vi "Enumerate Connected IMAQdx DirectShow Cameras.vi"() -> ()   [LabVIEW 2011]
uses:
  <vilib>/vision/driver/NI_Vision_Acquisition_Software.lvlib
panel:
  out "Connected Camera Interface name":string[](array[string])
  out "IMAQdx Open Camera error":errorcluster[](array[cluster])
  out "IMAQdx Enumerate Connected Only Cameras Camera Information Array":T1(array[cluster]) {"BusType" format="%x"; "SerialNumberLow" format="%.0x"; "SerialNumberHigh" format="%.0x"}
  # "Certain USB DirectShow cameras will always as connected when they are not.  Acording to one vendor :\n\"USB cameras that implement their DirectShow driver as a data source filter and register the filter as a \"video capture device\" \nwill always shows the device (filter) no matter whether the physical device is connected or not. \nThis contrasts with many other USB cameras (e.g. all web cameras) which implement their DirectShow support with a WDM stream driver.\""
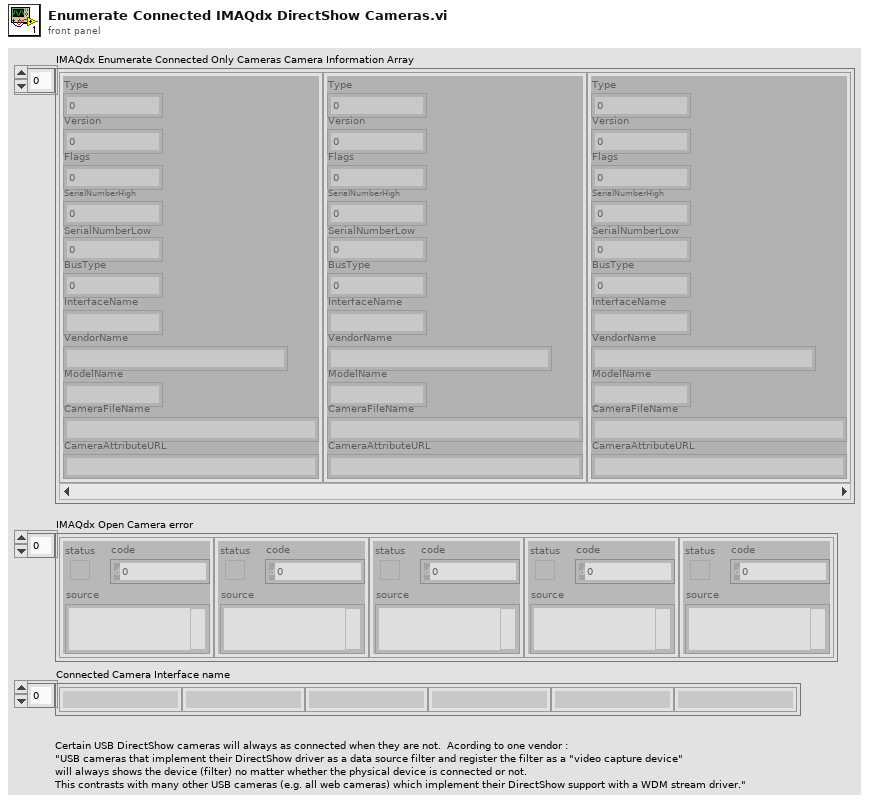
[diagram p1: front panel]
types:
  T1 = cluster{"Type":u32, "Version":u32, "Flags":u32, "SerialNumberHigh":u32, "SerialNumberLow":u32, "BusType":u32, "InterfaceName":string, "VendorName":string, "ModelName":string, "CameraFileName":string, "CameraAttributeURL":string}[]
  T2 = typedef "IMAQdx.ctl" = refnum<k21>
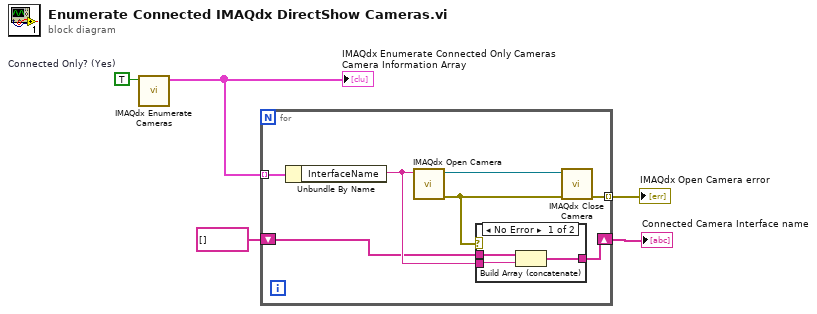
[diagram p0: block diagram]
diagram:
  w1 = TRUE  # Connected Only? (Yes)
  n1 = call <vilib>:"IMAQdx Enumerate Cameras.vi"("Connected Only? (Yes)"=w1) -> ("Camera Information Array"=w5:T1)  [unwired: 9 in, 1 out]
  "IMAQdx Enumerate Connected Only Cameras Camera Information Array" <- w5
  n2 = for {
    tunnel: w5 -> [w12] mode=indexing
    tunnel: [w10] -> w4 mode=indexing
    shift-right: [w7] -> w2
    shift-left: string[] [] -> [w6]
    n3 = Unbundle By Name(w12) -> ("InterfaceName"=w8:string)
    n4 = call <vilib>:"IMAQdx Open Camera.vi"("Session In"=w8) -> ("error out"=w9:errorcluster, "Session Out"=w11:T2)  [unwired: 9 in]
    n5 = case shown="No Error" w9 {
      tunnel: w8 -> [w15 _]
      tunnel: [w14 w16] -> w7
      tunnel: w6 -> [w13 w16]
      frame No Error {
        n6 = Build Array (concatenate)(w13, w15) -> (w14:string[])
      }
      frame Error {
      }
    }
    n7 = call <vilib>:"IMAQdx Close Camera.vi"("error in"=w9, "Session In"=w11) -> ("error out"=w10:errorcluster)  [unwired: 9 in]
  }
  "IMAQdx Open Camera error" <- w4
  "Connected Camera Interface name" <- w2
